vi "Strip Single Control.vi"(0 "Ctl Refnum":refnum<vi>, 1 "Cluster Refnum":refnum<vi>, 3 "Label.Text":string, 5 "Keys in":string[](array[string]), 7 "Values in":string[](array[string]), 9 "Formatting":T1, 11 "error in (no error)":errorcluster, 12 "Strip Cluster":refnum<vi>, 14 "Value":variant) -> (4 "Ctl Refnum":refnum<vi>, 6 "Keys out":string[](array[string]), 8 "Values out":string[](array[string]), 15 "error out":errorcluster)   [LabVIEW 2018]
uses:
  Cluster Formatting.ctl
panel:
  in  "type specifier":refnum<vi>
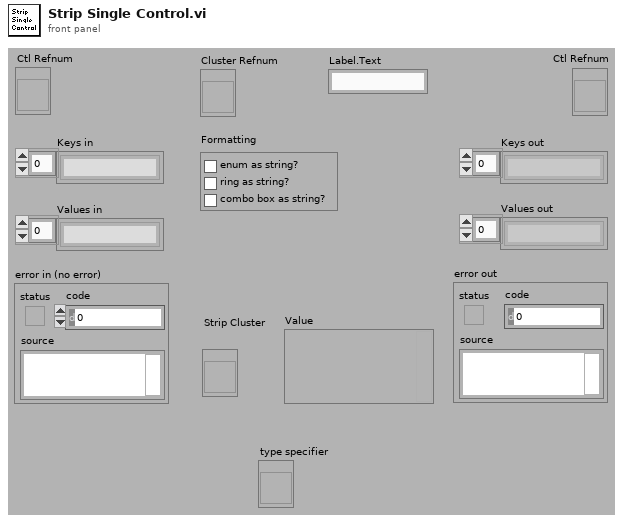
[diagram p1: front panel]
types:
  T1 = typedef "Cluster Formatting.ctl" = cluster{"enum as string?":bool, "ring as string?":bool, "combo box as string?":bool}
  T2 = typedef "LVComboBoxStrsAndValuesArrayTypeDef.ctl" = cluster{"String":string, "Value":string}[]
  T3 = typedef "LVStringsAndValuesArrayTypeDef.ctl" = cluster{"String":string, "Value":ext}[]
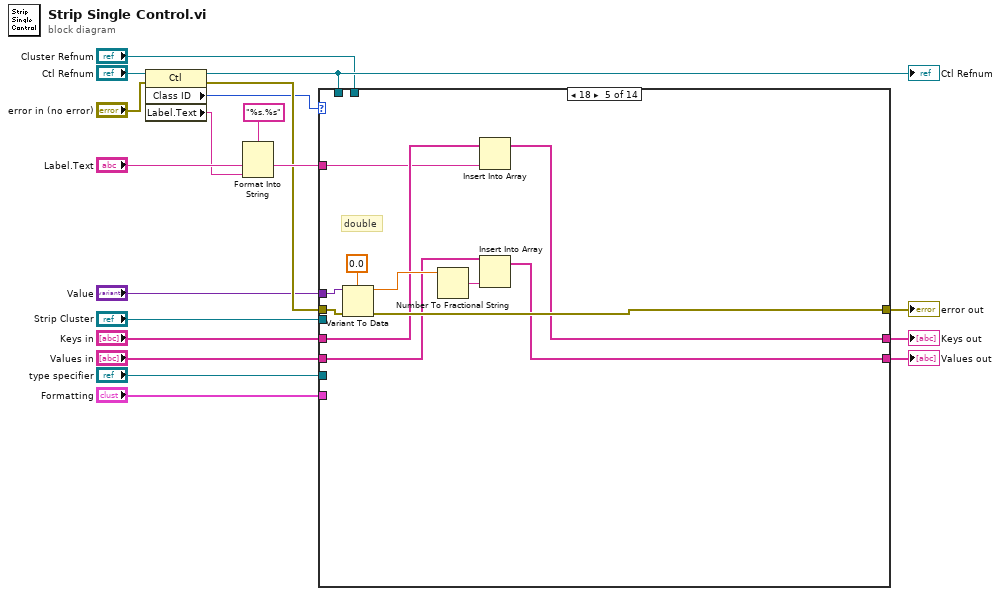
[diagram p0: block diagram]
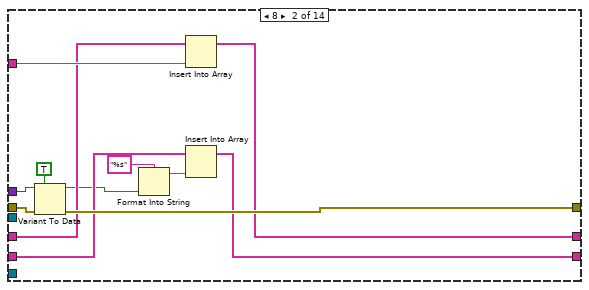
[diagram p3: hidden frame]
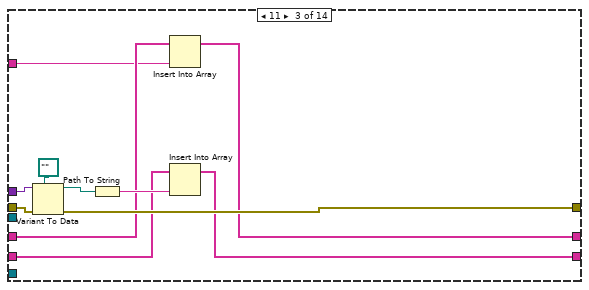
[diagram p4: hidden frame]
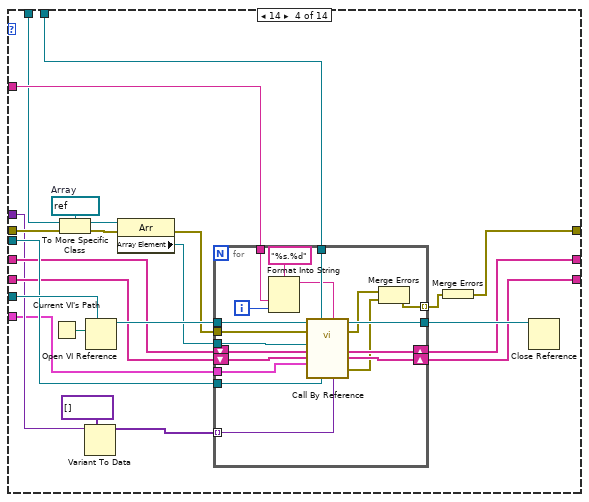
[diagram p5: hidden frame]
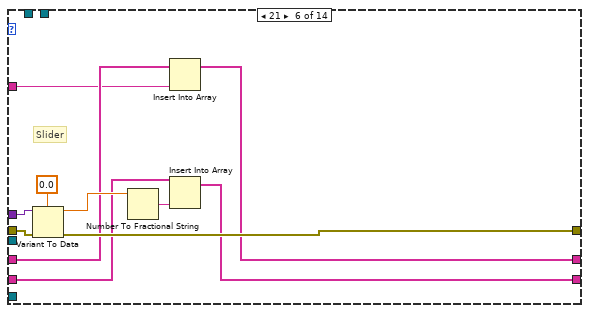
[diagram p6: hidden frame]
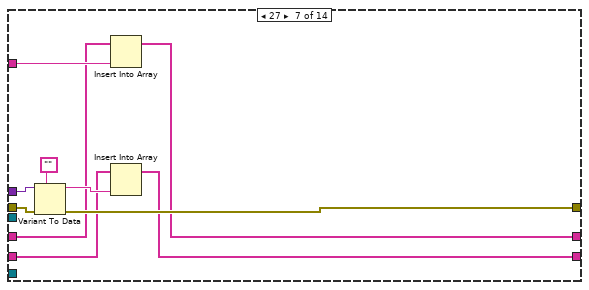
[diagram p7: hidden frame]
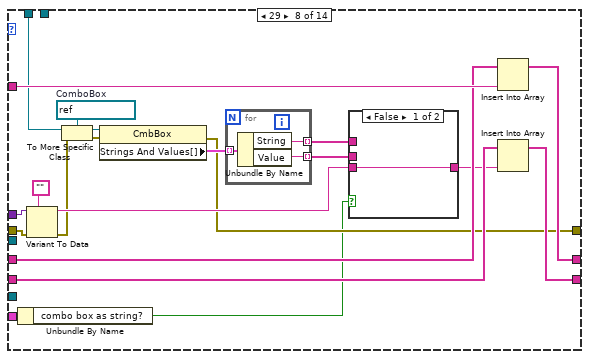
[diagram p8: hidden frame]
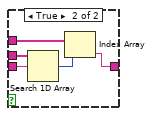
[diagram p9: hidden frame]
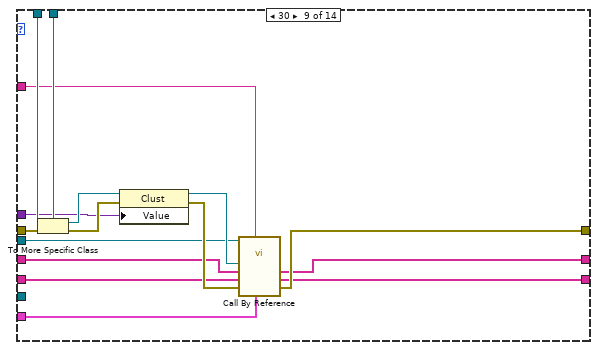
[diagram p10: hidden frame]
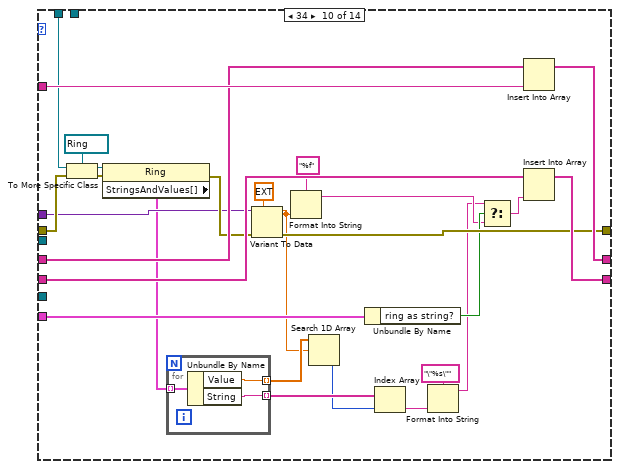
[diagram p11: hidden frame]
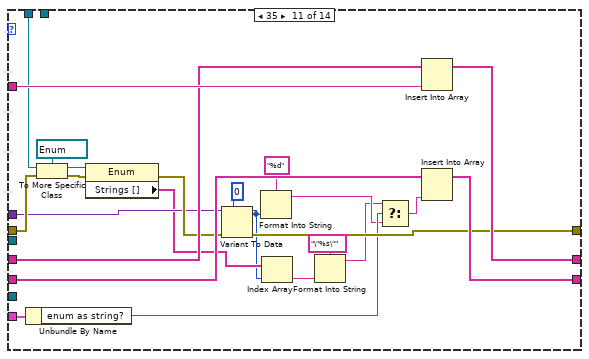
[diagram p12: hidden frame]
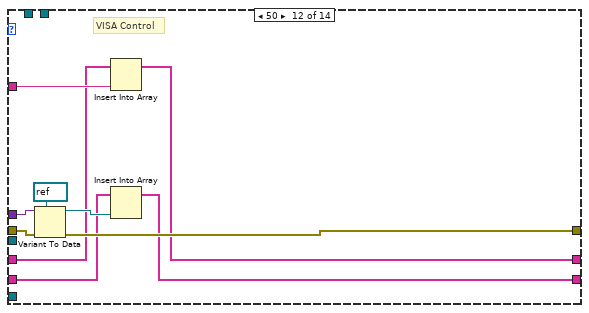
[diagram p13: hidden frame]
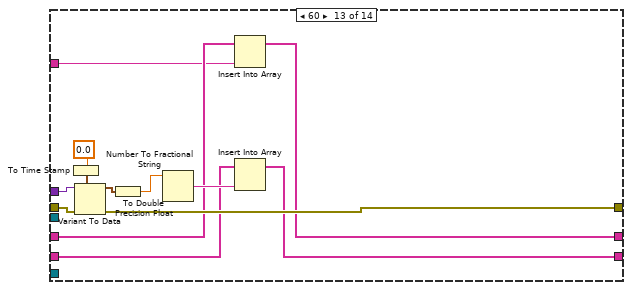
[diagram p14: hidden frame]
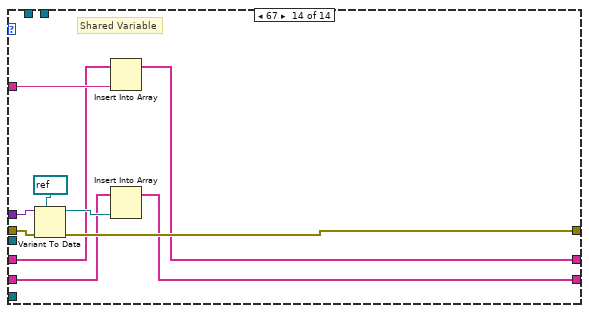
[diagram p15: hidden frame]
diagram:
  n1 = property class="Ctl"(reference="Ctl Refnum", error in="error in (no error)") -> (reference out=w18:refnum<vi>, error out=w9:errorcluster, "Class ID"=w6:u32, "Label.Text"=w17:string)
  "Ctl Refnum" <- w18
  n2 = Format Into String(format string="%s.%s", "Label.Text", w17) -> (resulting string=w12:string)  [unwired: 2 in, 1 out]
  n3 = case shown="18" w6 {
    tunnel: "Value" -> [_ w33 w45 w47 w99 w110 w120 w141 w161 w175 w202 w230 w243 w253]
    tunnel: w9 -> [w22 w34 w44 w48 w96 w107 w118 w125 w164 w186 w213 w229 w241 w252]
    tunnel: [w22 w32 w43 w50 w95 w106 w117 w123 w155 w181 w208 w228 w240 w251] -> w10
    tunnel: "Strip Cluster" -> [_ _ _ w65 _ _ _ _ w152 _ _ _ _ _]
    tunnel: "Cluster Refnum" -> [_ _ _ w56 _ _ _ _ w165 _ _ _ _ _]
    tunnel: w12 -> [_ w30 w37 w52 w91 w102 w114 w138 w156 w193 w220 w225 w233 w248]
    tunnel: [w21 w27 w36 w58 w90 w101 w112 w136 w153 w190 w217 w223 w232 w246] -> w15
    tunnel: "Keys in" -> [w21 w29 w38 w60 w92 w103 w113 w137 w158 w192 w219 w224 w234 w247]
    tunnel: "Values in" -> [w20 w28 w39 w59 w93 w104 w115 w139 w159 w191 w218 w226 w235 w249]
    tunnel: [w20 w26 w35 w57 w89 w100 w111 w135 w154 w189 w216 w222 w231 w245] -> w16
    tunnel: w18 -> [_ _ _ w49 _ _ _ w130 w166 w187 w214 _ _ _]
    tunnel: "type specifier" -> [_ _ _ w66 _ _ _ _ _ _ _ _ _ _]
    tunnel: "Formatting" -> [_ _ _ w46 _ _ _ w122 w151 w179 w206 _ _ _]
    frame 0, Default {
    }
    frame 8 {
      n4 = Variant To Data(error in=w34, type=TRUE, Variant=w33) -> (data=w24:bool, error out=w32:errorcluster)
      n5 = Format Into String(format string="%s", w24) -> (resulting string=w23:string)  [unwired: 2 in, 1 out]
      n6 = Insert Into Array(array=w29, new element=w30) -> (w27:string[])  [unwired: 1 in]
      n7 = Insert Into Array(array=w28, new element=w23) -> (w26:string[])  [unwired: 1 in]
    }
    frame 11 {
      n8 = Variant To Data(error in=w44, type=path "", Variant=w45) -> (data=w41:path, error out=w43:errorcluster)
      n9 = Path To String(path=w41) -> (string=w40:string)
      n10 = Insert Into Array(array=w38, new element=w37) -> (w36:string[])  [unwired: 1 in]
      n11 = Insert Into Array(array=w39, new element=w40) -> (w35:string[])  [unwired: 1 in]
    }
    frame 14 {
      w64 = refnum<vi> refnum  # Array
      n12 = Current VI's Path() -> (path=w69:path)
      n13 = To More Specific Class(target class=w64, reference=w49, error in=w48) -> (specific class reference=w63:refnum<vi>, error out=w62:errorcluster)
      n14 = Variant To Data(type=variant[] [], Variant=w47) -> (data=w54:variant[])  [unwired: 1 in, 1 out]
      n15 = Open VI Reference(type specifier VI Refnum (for type only)=w66, vi path=w69) -> (vi reference=w68:refnum<vi>)  [unwired: 4 in, 1 out]
      n16 = property class="Arr"(reference=w63, error in=w62) -> (error out=w55:errorcluster, "Array Element"=w61:refnum<vi>)  [unwired: 1 out]
      n17 = for {
        tunnel: w68 -> [w88]
        tunnel: [w87] -> w67
        tunnel: w65 -> [w86]
        tunnel: w61 -> [w85]
        tunnel: w56 -> [w80]
        shift-right: [w82] -> w58
        shift-left: w60 -> [w84]
        shift-right: [w81] -> w57
        shift-left: w59 -> [w83]
        tunnel: w55 -> [w79]
        tunnel: w54 -> [w71] mode=indexing
        tunnel: w52 -> [w77]
        tunnel: [w72] -> w51 mode=indexing
        tunnel: w46 -> [w70]
        i -> [w76]
        n18 = Format Into String(format string="%s.%d", w77, w76) -> (resulting string=w75:string)  [unwired: 2 in, 1 out]
        n19 = call-by-ref "?"(reference=w88, error in=w79, "Ctl Refnum"=w85, "Cluster Refnum"=w80, "Label.Text"=w75, "Keys in"=w84, "Values in"=w83, "Formatting"=w70, "Strip Cluster"=w86, "Value"=w71) -> (reference out=w87:refnum<vi>, error out=w74:errorcluster, "Keys out"=w82:string[], "Values out"=w81:string[], 15:"error out"=w73:errorcluster)  [unwired: 4 in, 1 out]
        n20 = Merge Errors(w74, w73) -> (w72:errorcluster)
      }
      n21 = Merge Errors(w51) -> (w50:errorcluster)
      n22 = Close Reference(reference=w67) -> ()  [unwired: 1 in, 1 out]
    }
    frame 18 {
      # "double"
      n23 = Variant To Data(error in=w96, type=0.0, Variant=w99) -> (data=w97:dbl, error out=w95:errorcluster)
      n24 = Number To Fractional String(number=w97) -> (F-format string=w94:string)  [unwired: 3 in]
      n25 = Insert Into Array(array=w92, new element=w91) -> (w90:string[])  [unwired: 1 in]
      n26 = Insert Into Array(array=w93, new element=w94) -> (w89:string[])  [unwired: 1 in]
    }
    frame 21 {
      # "Slider"
      n27 = Variant To Data(error in=w107, type=0.0, Variant=w110) -> (data=w108:dbl, error out=w106:errorcluster)
      n28 = Number To Fractional String(number=w108) -> (F-format string=w105:string)  [unwired: 3 in]
      n29 = Insert Into Array(array=w103, new element=w102) -> (w101:string[])  [unwired: 1 in]
      n30 = Insert Into Array(array=w104, new element=w105) -> (w100:string[])  [unwired: 1 in]
    }
    frame 27 {
      n31 = Variant To Data(error in=w118, type="", Variant=w120) -> (data=w116:string, error out=w117:errorcluster)
      n32 = Insert Into Array(array=w113, new element=w114) -> (w112:string[])  [unwired: 1 in]
      n33 = Insert Into Array(array=w115, new element=w116) -> (w111:string[])  [unwired: 1 in]
    }
    frame 29 {
      w134 = refnum<vi> refnum  # ComboBox
      n34 = Unbundle By Name(w122) -> ("combo box as string?"=w121:bool)
      n35 = Variant To Data(error in=w125, type="", Variant=w141) -> (data=w127:string, error out=w124:errorcluster)
      n36 = To More Specific Class(target class=w134, reference=w130, error in=w124) -> (specific class reference=w133:refnum<vi>, error out=w132:errorcluster)
      n37 = property class="CmbBox"(reference=w133, error in=w132) -> (error out=w123:errorcluster, "Strings And Values[]"=w131:T2)  [unwired: 1 out]
      n38 = for {
        tunnel: w131 -> [w150] mode=indexing
        tunnel: [w149] -> w129 mode=indexing
        tunnel: [w148] -> w128 mode=indexing
        n39 = Unbundle By Name(w150) -> ("String"=w148:string, "Value"=w149:string)
      }
      n40 = case shown="False" w121 {
        tunnel: w129 -> [_ w147]
        tunnel: w127 -> [w142 w146]
        tunnel: w128 -> [_ w145]
        tunnel: [w142 w143] -> w126
        frame False {
        }
        frame True {
          n41 = Search 1D Array(1D array=w147, element=w146) -> (index of element=w144:i32)  [unwired: 1 in]
          n42 = Index Array(array=w145, index=w144) -> (element=w143:string)
        }
      }
      n43 = Insert Into Array(array=w137, new element=w138) -> (w136:string[])  [unwired: 1 in]
      n44 = Insert Into Array(array=w139, new element=w126) -> (w135:string[])  [unwired: 1 in]
    }
    frame 30 {
      n45 = To More Specific Class(target class=w165, reference=w166, error in=w164) -> (specific class reference=w163:refnum<vi>, error out=w162:errorcluster)
      n46 = property class="Clust"(reference=w163, error in=w162, "Value"=w161) -> (reference out=w157:refnum<vi>, error out=w160:errorcluster)
      n47 = call-by-ref "?"(reference=w152, "Configuration"=w151, "Prefix Name"=w156, "error in (no error)"=w160, "Values in"=w159, "Key in"=w158, "Cluster Refnum"=w157) -> ("error out"=w155:errorcluster, "Values"=w154:string[], "Keys"=w153:string[])  [unwired: 3 in, 3 out]
    }
    frame 34 {
      n48 = To More Specific Class(target class=refnum<vi> refnum ("Enum Class"), reference=w187, error in=w186) -> (specific class reference=w185:refnum<vi>, error out=w184:errorcluster)
      n49 = property class="Ring"(reference=w185, error in=w184) -> (error out=w182:errorcluster, "StringsAndValues[]"=w171:T3)  [unwired: 1 out]
      n50 = for {
        tunnel: w171 -> [w196] mode=indexing
        tunnel: [w195] -> w169 mode=indexing
        tunnel: [w194] -> w170 mode=indexing
        n51 = Unbundle By Name(w196) -> ("Value"=w194:ext, "String"=w195:string)
      }
      n52 = Variant To Data(error in=w182, type=ext 0.0 ("unsigned 32bit integer"), Variant=w175) -> (data=w168:ext, error out=w181:errorcluster)
      n53 = Format Into String(format string="%f", w168) -> (resulting string=w177:string)  [unwired: 2 in, 1 out]
      n54 = Search 1D Array(1D array=w170, element=w168) -> (index of element=w167:i32)  [unwired: 1 in]
      n55 = Unbundle By Name(w179) -> ("ring as string?"=w178:bool)
      n56 = Index Array(array=w169, index=w167) -> (element=w174:string)
      n57 = Format Into String(format string="\"%s\"", w174) -> (resulting string=w173:string)  [unwired: 2 in, 1 out]
      n58 = Select(t=w173, s=w178, f=w177) -> (s? t:f=w176:string)
      n59 = Insert Into Array(array=w192, new element=w193) -> (w190:string[])  [unwired: 1 in]
      n60 = Insert Into Array(array=w191, new element=w176) -> (w189:string[])  [unwired: 1 in]
    }
    frame 35 {
      n61 = Unbundle By Name(w206) -> ("enum as string?"=w205:bool)
      n62 = To More Specific Class(target class=refnum<vi> refnum ("Enum Class"), reference=w214, error in=w213) -> (specific class reference=w212:refnum<vi>, error out=w211:errorcluster)
      n63 = property class="Enum"(reference=w212, error in=w211) -> (error out=w209:errorcluster, "Strings []"=w201:string[])  [unwired: 1 out]
      n64 = Variant To Data(error in=w209, type=u32 0 ("unsigned 32bit integer"), Variant=w202) -> (data=w200:u32, error out=w208:errorcluster)
      n65 = Format Into String(format string="%d", w200) -> (resulting string=w204:string)  [unwired: 2 in, 1 out]
      n66 = Index Array(array=w201, index=w200) -> (element=w199:string)
      n67 = Format Into String(format string="\"%s\"", w199) -> (resulting string=w198:string)  [unwired: 2 in, 1 out]
      n68 = Select(t=w198, s=w205, f=w204) -> (s? t:f=w203:string)
      n69 = Insert Into Array(array=w219, new element=w220) -> (w217:string[])  [unwired: 1 in]
      n70 = Insert Into Array(array=w218, new element=w203) -> (w216:string[])  [unwired: 1 in]
    }
    frame 50 {
      # "VISA Control"
      n71 = Variant To Data(error in=w229, type=refnum<visa-resource-name> refnum ("VISA resource name"), Variant=w230) -> (data=w227:refnum<visa-resource-name>, error out=w228:errorcluster)
      n72 = Insert Into Array(array=w224, new element=w225) -> (w223:string[])  [unwired: 1 in]
      n73 = Insert Into Array(array=w226, new element=w227) -> (w222:string[])  [unwired: 1 in]
    }
    frame 60 {
      n74 = To Time Stamp(1:0.0) -> (0:w238:timestamp)
      n75 = Variant To Data(error in=w241, type=w238, Variant=w243) -> (data=w242:timestamp, error out=w240:errorcluster)
      n76 = To Double Precision Float(number=w242) -> (double precision float=w237:dbl)
      n77 = Number To Fractional String(number=w237) -> (F-format string=w236:string)  [unwired: 3 in]
      n78 = Insert Into Array(array=w234, new element=w233) -> (w232:string[])  [unwired: 1 in]
      n79 = Insert Into Array(array=w235, new element=w236) -> (w231:string[])  [unwired: 1 in]
    }
    frame 67 {
      # "Shared Variable"
      n80 = Variant To Data(error in=w252, type=refnum<k21> refnum, Variant=w253) -> (data=w250:refnum<k21>, error out=w251:errorcluster)
      n81 = Insert Into Array(array=w247, new element=w248) -> (w246:string[])  [unwired: 1 in]
      n82 = Insert Into Array(array=w249, new element=w250) -> (w245:string[])  [unwired: 1 in]
    }
  }
  "Values out" <- w16
  "Keys out" <- w15
  "error out" <- w10
